vi "FindLeakMapCoordinate.vi"(4 "Y":dbl[](array[numeric]), 5 "Z":dbl[](array[numeric]), 6 "reference 4":refnum<vi>, 7 "X":dbl[](array[numeric]), 9 "reference 3":refnum<vi>, 10 "reference输入":refnum<vi>, 11 "String输入":refnum<vi>) -> (2 "X":string, 3 "Y":string)   [LabVIEW 2014, in "cyy.lvlib" / "LeakageFenXi.lvlib"]
uses:
  LeakageFenXi.lvlib
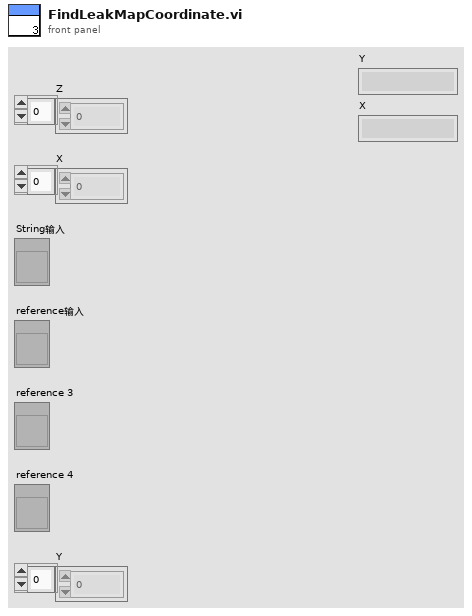
[diagram p1: front panel]
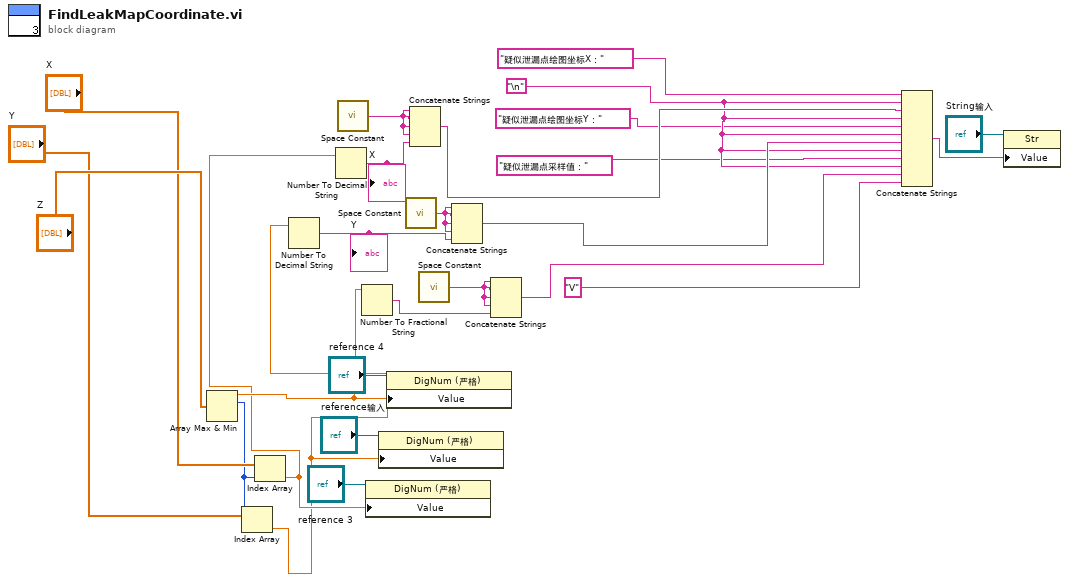
[diagram p0: block diagram]
diagram:
  w12 = "\n"
  n1 = Array Max & Min(array="Z") -> (max value=w26:dbl, max index (indices)=w5:i32)  [unwired: 2 out]
  n2 = Index Array(array="Y", index=w5) -> (element=w24:dbl)
  n3 = Index Array(array="X", index=w5) -> (element=w25:dbl)
  n4 = Number To Decimal String(number=w24) -> (decimal integer string=w18:string)  [unwired: 1 in]
  "Y" <- w18
  n5 = Number To Decimal String(number=w25) -> (decimal integer string=w15:string)  [unwired: 1 in]
  "X" <- w15
  n6 = call <vilib>:"Space Constant.vi"() -> ("String"=w14:string)
  n7 = Number To Fractional String(number=w26) -> (F-format string=w21:string)  [unwired: 3 in]
  n8 = property class="DigNum (严格)"(reference="reference 3", "Value"=w25) -> ()  [unwired: 1 in, 2 out]
  n9 = property class="DigNum (严格)"(reference="reference输入", "Value"=w24) -> ()  [unwired: 1 in, 2 out]
  n10 = property class="DigNum (严格)"(reference="reference 4", "Value"=w26) -> ()  [unwired: 1 in, 2 out]
  n11 = call <vilib>:"Space Constant.vi"() -> ("String"=w17:string)
  n12 = Concatenate Strings(w14, w14, w14, w14, w15) -> (w16:string)
  n13 = call <vilib>:"Space Constant.vi"() -> ("String"=w20:string)
  n14 = Concatenate Strings(w17, w17, w17, w17, w18) -> (w19:string)
  n15 = Concatenate Strings(w20, w20, w20, w20, w21) -> (w22:string)
  n16 = Concatenate Strings("疑似泄漏点绘图坐标X：", w12, w16, w12, "疑似泄漏点绘图坐标Y：", w12, w19, w12, "疑似泄漏点采样值：", w12, w22, "V") -> (w23:string)
  n17 = property class="Str"(reference="String输入", "Value"=w23) -> ()  [unwired: 1 in, 2 out]
